vi "List Windows Application.vi"() -> ()   [LabVIEW 2019, in "Tools.lvlib"]
uses:
  Tools.lvlib
panel:
  out "Names of Application Windows":string[](array[string])
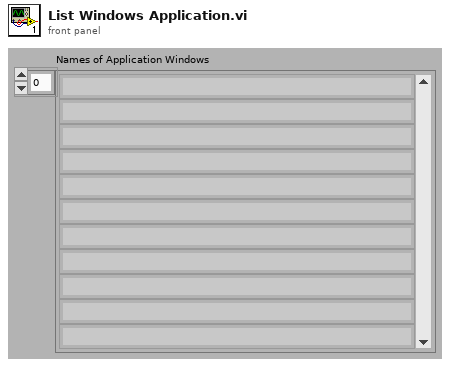
[diagram p1: front panel]
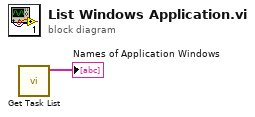
[diagram p0: block diagram]
diagram:
  n1 = call "Get Task List.vi"() -> ("names of application windows"=→"Names of Application Windows":string[])  [unwired: 6 in, 1 out]
